vi "Release.vi"(8 "error in (no error)":errorcluster, 11 "IContainersNotiferOrEvents in":refnum<class "IContainersNotiferOrEvents.lvclass">) -> (0 "error out":errorcluster)   [LabVIEW 2020, in "wamplv.lvlib" / "IContainersNotiferOrEvents.lvclass"]
uses:
  IContainersNotiferOrEvents.lvclass
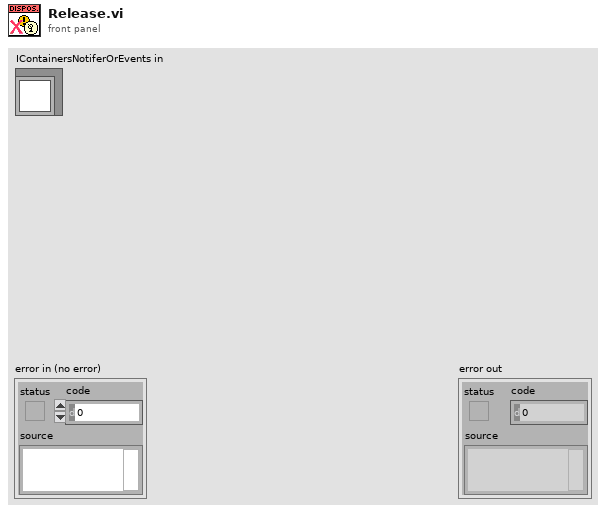
[diagram p1: front panel]
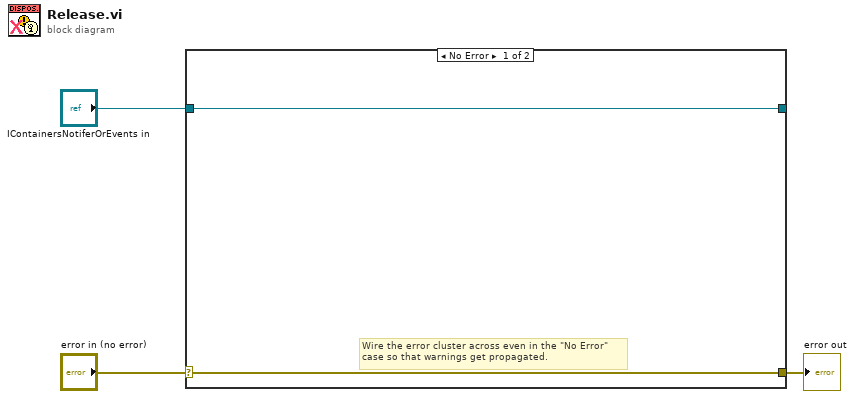
[diagram p0: block diagram]
diagram:
  n1 = case shown="No Error" "error in (no error)" {
    selector: "error in (no error)" -> [w4 w7]
    tunnel: [w4 w7] -> w2
    tunnel: [w5 w6] -> _
    tunnel: "IContainersNotiferOrEvents in" -> [w5 w6]
    frame No Error {
      # "Wire the error cluster across even in the \"No Error\"\ncase so that warnings get propagated."
    }
    frame Error {
    }
  }
  "error out" <- w2
